vi "Create.vi"(10 "Channel":refnum<class "Channel DBL.lvclass">) -> (3 "ChannelValue out":refnum<class "DoubleChannelValue.lvclass">)   [LabVIEW 2020, in "Vecto.lvlib" / "DoubleChannelValue.lvclass"]
uses:
  DoubleChannelValue.lvclass
  Channel DBL/Channel DBL.lvclass
  DoubleChannelValue.lvclass/DoubleChannelValue.ctl
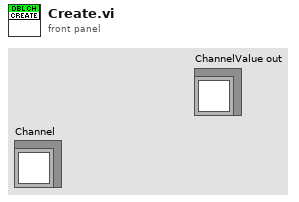
[diagram p1: front panel]
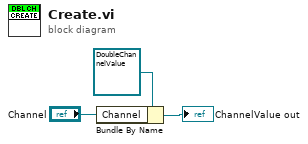
[diagram p0: block diagram]
diagram:
  n1 = Bundle By Name(cluster=refnum<class "DoubleChannelValue.lvclass"> refnum ("ChannelValue in"), "Channel"="Channel") -> (→"ChannelValue out":refnum<class "DoubleChannelValue.lvclass">)
